vi "Logic_Add_SPI_Analyzer.vi"(4 "error in (no error)":errorcluster, 5 "Analyzer Settings":T1={"MOSI Channel"=0, "MISO Channel"=1, "CLOCK Channel"=2, "ENABLE Channel"=3, "Bits per Transfer"="8 Bits per Transfer (Standard)"}, 6 "Analyzer Label":string="Test Analyzer", 7 "Session Ref In":T2) -> (0 "error out":errorcluster, 1 "Debug Status":string, 3 "Session Ref Out":T2)   [LabVIEW 2023]
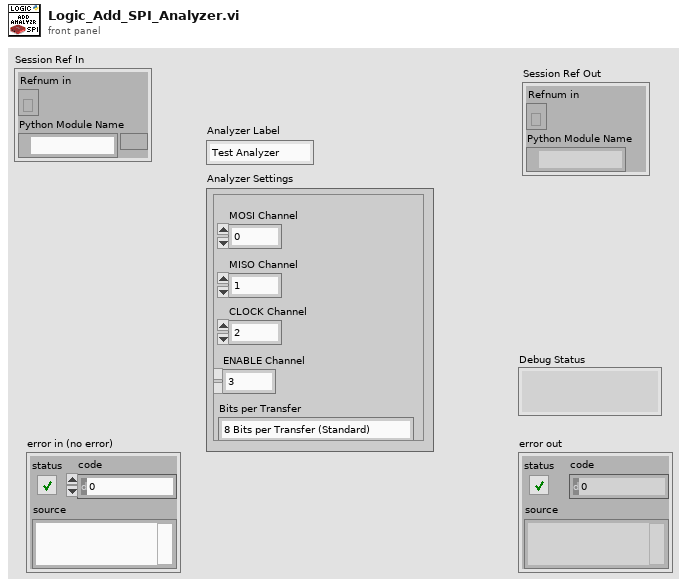
[diagram p1: front panel]
types:
  T1 = cluster{"MOSI Channel":i32, "MISO Channel":i32, "CLOCK Channel":i32, "ENABLE Channel":i32, "Bits per Transfer":string}
  T2 = cluster{"Refnum in":refnum<k35>, "Python Module Name":path}
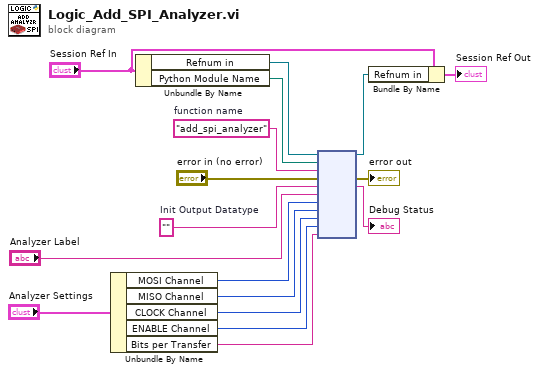
[diagram p0: block diagram]
diagram:
  w15 = "add_spi_analyzer"  # function name
  w14 = ""  # Init Output Datatype
  n1 = Unbundle By Name("Analyzer Settings") -> ("MOSI Channel"=w6:i32, "MISO Channel"=w5:i32, "CLOCK Channel"=w4:i32, "ENABLE Channel"=w3:i32, "Bits per Transfer"=w2:string)
  n2 = Unbundle By Name("Session Ref In") -> ("Refnum in"=w12:refnum<k35>, "Python Module Name"=w11:path)
  n3 = node(w12, w11, w15, "error in (no error)", w14, "Analyzer Label", w6, w5, w4, w3, w2) -> (w9:refnum<k35>, →"error out":errorcluster, →"Debug Status":string)  [unwired: 6 in, 2 out]
  n4 = Bundle By Name(cluster="Session Ref In", "Refnum in"=w9) -> (→"Session Ref Out":T2)
